vi "Read Image File Directory.vi"(2 "Im_File_Dir Offs":i32, 3 "Image Data in":u8[](array[numeric])) -> (0 "Directory":T1[](array[typedef]), 1 "Image Data out":u8[](array[numeric]))   [LabVIEW 2014, in "LAVA TIFF File Reader.lvlib"]
doc: "Reads the tags and associated data in a tiff file byte stream (Image Data in) starting at an offset (Image File Directory Offset) which is determined using the Read Header.vi. Returns an array of clusters containing the tag and location and format of the assocaited data."
uses:
  LAVA TIFF File Reader.lvlib
  TypeDefs/IFD Entry.ctl
  TypeDefs/FieldTypes.ctl
panel:
  out "Numeric":i32
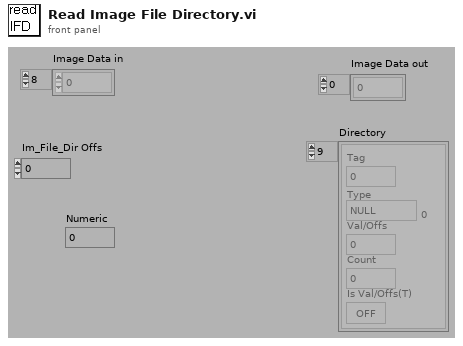
[diagram p1: front panel]
types:
  T1 = typedef "LAVA TIFF File Reader.lvlib/IFD Entry.ctl" = cluster{"Tag":u16, "Type":T2, "Count":u32, "Val/Offs":u32, "Is Val/Offs(T)":bool}
  T2 = typedef "LAVA TIFF File Reader.lvlib/FieldTypes.ctl" = enum16{"NULL", "U8", "ASCII7", "U16", "U32", "RATIONAL", "SByte(I8)", "Undef(8Bit)", "I16", "I32", "SRat(4B:4B)", "SGL(4Byte)", "DBL(8Byte)"}
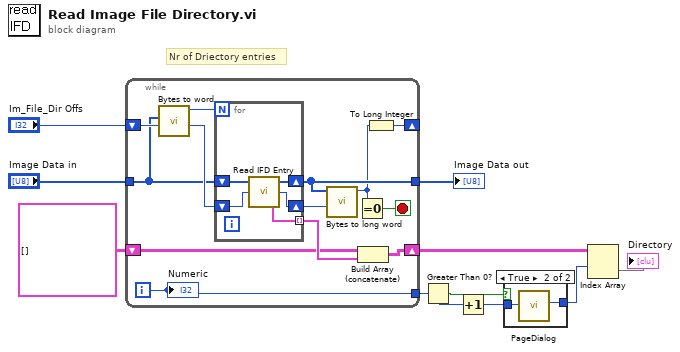
[diagram p0: block diagram]
diagram:
  # "Nr of Driectory entries"
  n1 = while {
    tunnel: "Image Data in" -> [w13]
    tunnel: [w21] -> w8
    shift-right: [w14] -> _
    shift-left: "Im_File_Dir Offs" -> [w23]
    shift-right: [w16] -> w5
    shift-left: T1[][] [] -> [w17]
    tunnel: [w11] -> w1
    i -> [w11]
    stop <- w19 stop-if-true
    n2 = call "Bytes to word.vi"("Index"=w23, "Image Data in"=w13) -> ("Index+2"=w22:i32, "Word"=w12:u16)  [unwired: 6 in]
    n3 = for {
      N: w12 -> [_]
      shift-right: [w26] -> w21
      shift-left: w13 -> [w27]
      shift-right: [w25] -> w20
      shift-left: w22 -> [w28]
      tunnel: [w24] -> w18 mode=indexing
      n4 = call "Read IFD Entry.vi"("Directory Offset in"=w28, "Image Data in"=w27) -> ("Cluster"=w24:T1, "Directory Offset Out"=w25:i32, "Image Data Out"=w26:u8[])  [unwired: 1 in]
    }
    n5 = call "Bytes to long word.vi"("Index"=w20, "Image Data in"=w21) -> ("U32"=w15:u32)  [unwired: 6 in, 1 out]
    n6 = Equal To 0?(x=w15) -> (x = 0?=w19:bool)
    n7 = Build Array (concatenate)(w17, w18) -> (w16:T1[][])
    n8 = To Long Integer(number=w15) -> (32bit integer=w14:i32)
    "Numeric" <- w11
  }
  "Image Data out" <- w8
  n9 = Greater Than 0?(x=w1) -> (x > 0?=w6:bool)
  n10 = Increment(x=w1) -> (x+1=w2:i32)
  n11 = case shown="True" w6 {
    tunnel: w2 -> [_ w30]
    tunnel: [_ w29] -> w4
    frame False {
    }
    frame True {
      n12 = call "PageDialog.vi"("Nr of Pages"=w30) -> ("OpenPage.."=w29:u16)  [unwired: 10 in]
    }
  }
  n13 = Index Array(array=w5, index (row)=w4) -> (element=→"Directory":T1[])  [unwired: 1 in]
